vi "4b.vi"() -> ()   [LabVIEW 2015]
panel:
  out "Waveform Graph":dbl[][](graph)
  in  "Cluster":cluster{"Array":dbl[][]}
  in  "physical channels":tag="Dev1/ai0:2"
  in  "# of samples/channel":i32=1000
  in  "Sampling rate":dbl=10000.0
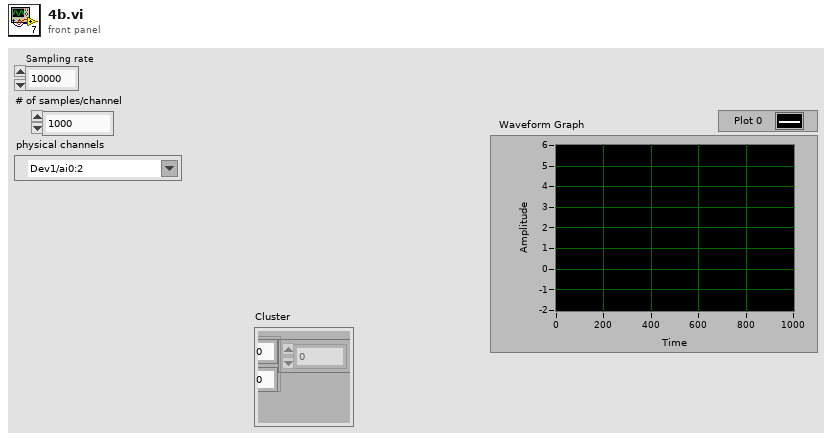
[diagram p1: front panel]
types:
  T1 = enum16{"open", "replace", "create", "open or create", "replace or create", "replace or create with confirmation"}
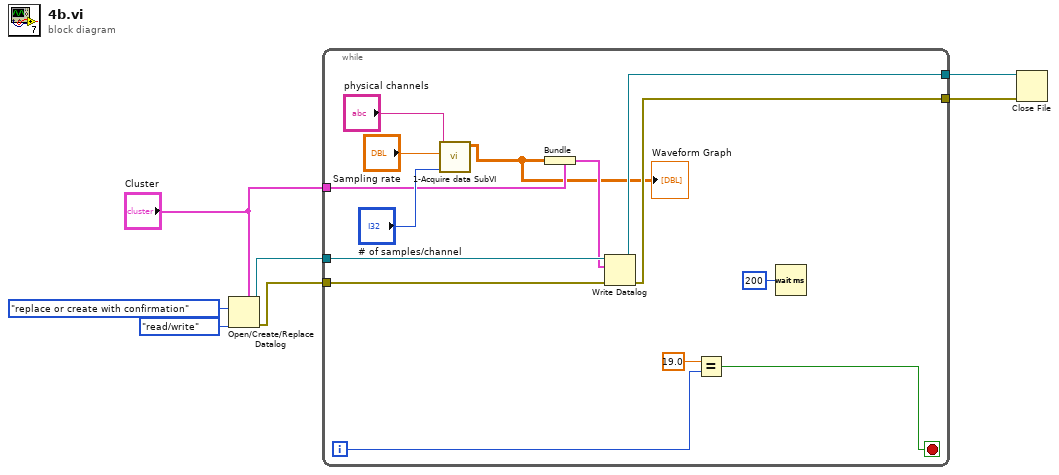
[diagram p0: block diagram]
diagram:
  n1 = Open/Create/Replace Datalog(5:"Cluster", 9:enum16{"read/write", "read-only", "write-only"}."read/write" ("access (0:read/write)"), 10:T1."replace or create with confirmation" ("operation (0:open)")) -> (0:w5:errorcluster, 3:w3:refnum<k1>)  [unwired: 3 in, 1 out]
  n2 = while {
    tunnel: w5 -> [w18]
    tunnel: [w17] -> w4
    tunnel: w3 -> [w16]
    tunnel: [w15] -> w2
    tunnel: "Cluster" -> [w14]
    i -> [w10]
    stop <- w9 stop-if-true
    n3 = call "1-Acquire data SubVI.vi"("# of samples/channel"="# of samples/channel", "Sampling rate"="Sampling rate", "physical channels"="physical channels") -> ("data"=w8:dbl[][])  [unwired: 8 in]
    "Waveform Graph" <- w8
    n4 = Bundle(cluster=w14, "Array"=w8) -> (w13:cluster{"Array":dbl[][]})
    n5 = Write Datalog(4:w18, 6:w13, 7:w16) -> (0:w17:errorcluster, 3:w15:refnum<k1>)
    n6 = Equal?(x=19.0, y=w10) -> (x = y?=w9:bool)
    n7 = Wait (ms)(milliseconds to wait=u32 200) -> ()  [unwired: 1 out]
  }
  n8 = Close File(refnum=w2, error in=w4) -> ()  [unwired: 2 out]
